vi "conv.Disabled.vi"(9 "NewVal":bool) -> (1 "f":T1(ring))   [LabVIEW 2020]
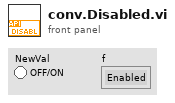
[diagram p1: front panel]
types:
  T1 = enum8{"Enabled", "Disabled", "Disabled and Grayed Out"}
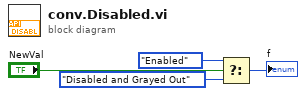
[diagram p0: block diagram]
diagram:
  n1 = Select(t=T1."Enabled" ("Disabled"), s="NewVal", f=T1."Disabled and Grayed Out") -> (s? t:f=→"f":T1)
